vi "Fail If Matching String.vi"(7 "Description":string, 8 "error in (no error)":errorcluster, 9 "Regular Expression":string, 10 "String":string, 11 "LUnit Test Case In":refnum<class "LUnit Test Case.lvclass">) -> (0 "error out":errorcluster, 3 "LUnit Test Case Out":refnum<class "LUnit Test Case.lvclass">)   [LabVIEW 2020, in "Advanced Assertions.lvlib"]
doc: "Generates a fail result for the calling test method if the String input contains a string which matches the given Regular Expression. The matching logic is the same as the LabVIEW native Match Pattern function. A description may be provided to the result."
uses:
  Advanced Assertions.lvlib
  LUnit Test Case/LUnit Test Case.lvclass
  LUnit Test Case/LUnit Test Case.lvclass/LUnit Test Case.ctl
  LUnit Test Case/Private/Append Pass Result.vi
  LUnit Test Case/Private/Append Fail Result.vi
  LUnit Test Case/Private/Run In UI.vi
  <vilib>/Utility/error.llb/Clear Errors.vi
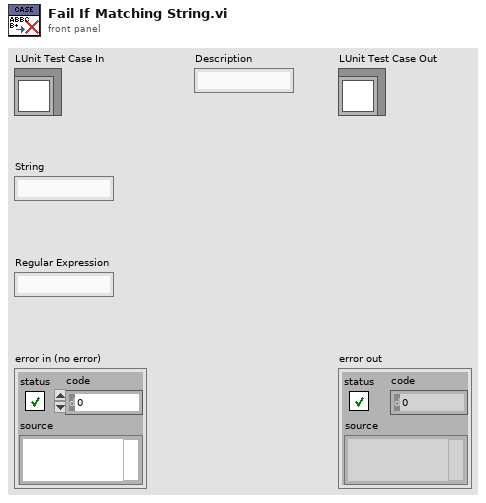
[diagram p1: front panel]
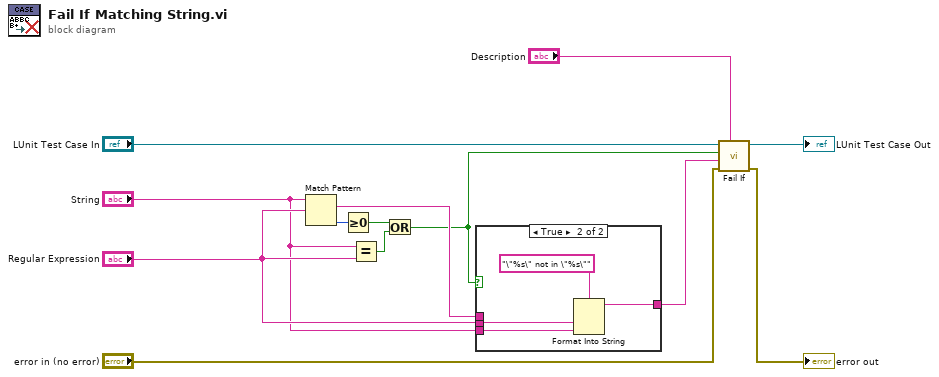
[diagram p0: block diagram]
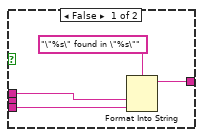
[diagram p2: hidden frame]
diagram:
  n1 = Match Pattern(string="String", regular expression="Regular Expression") -> (match substring=w3:string, offset past match=w8:i32)  [unwired: 1 in, 2 out]
  n2 = Greater Or Equal To 0?(x=w8) -> (x >= 0?=w7:bool)
  n3 = Equal?(x="String", y="Regular Expression") -> (x = y?=w6:bool)
  n4 = Or(x=w7, y=w6) -> (x .or. y?=w2:bool)
  n5 = case shown="True" w2 {
    tunnel: "Regular Expression" -> [_ w20]
    tunnel: "String" -> [w16 w19]
    tunnel: w3 -> [w15 _]
    tunnel: [w14 w18] -> w1
    frame False {
      n6 = Format Into String(format string="\"%s\" found in \"%s\"", w15, w16) -> (resulting string=w14:string)  [unwired: 2 in, 1 out]
    }
    frame True {
      n7 = Format Into String(format string="\"%s\" not in \"%s\"", w20, w19) -> (resulting string=w18:string)  [unwired: 2 in, 1 out]
    }
  }
  n8 = call "Fail If.vi"("Description"="Description", "error in (no error)"="error in (no error)", "Message"=w1, "Fail?"=w2, "LUnit Test Case In"="LUnit Test Case In") -> ("error out"=→"error out":errorcluster, "LUnit Test Case Out"=→"LUnit Test Case Out":refnum<class "LUnit Test Case.lvclass">)  [unwired: 5 in]
